vi "Load Module.vi"(8 "error in":errorcluster) -> (0 "error out":errorcluster)   [LabVIEW 2020, in "DBModule.lvlib"]
doc: "____\nHAMPEL SOFTWARE ENGINEERING v2.6.0 (2023-12-19 10:54)"
uses:
  DBModule.lvlib
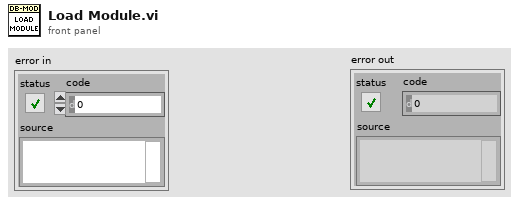
[diagram p1: front panel]
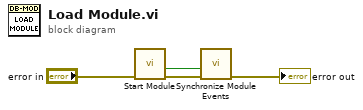
[diagram p0: block diagram]
diagram:
  n1 = call "Start Module.vi"("error in (no error)"="error in") -> ("error out"=w3:errorcluster, "Wait for Event Sync?"=w4:bool)  [unwired: 7 in, 2 out]
  n2 = call "Synchronize Module Events.vi"("error in (no error)"=w3, "Wait for Event Sync?"=w4) -> ("error out"=→"error out":errorcluster)  [unwired: 9 in]
